vi "UDSSetGenealogy.vi"(8 "Error In":errorcluster, 9 "DataToSet":string[](array[string]), 10 "GenealogyItemsToSet":T1[](array[typedef]), 11 "SessionID":string) -> (0 "Error Out":errorcluster, 2 "Success?":bool)   [LabVIEW 2021, in "Lunar UDS CAN.lvlib"]
uses:
  Lunar UDS CAN.lvlib
  Controls/UDSGenealogyItems.ctl
  Controls/UDSActions.ctl
  abd07550-7e02-4878-985a-2b81226fabe2.vi
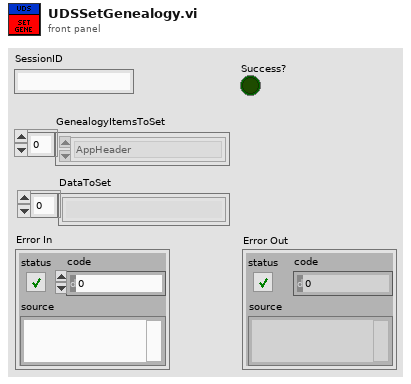
[diagram p1: front panel]
types:
  T1 = typedef "Lunar UDS CAN.lvlib/UDSGenealogyItems.ctl" = enum16{"AppHeader", "Genealogy Block Init", "Genealogy Block", "Board Part Number", "Board Serial Number", "Aux1 Part Number", "Aux1 Serial Number", "Aux2 Part Number", "Aux2 Serial Number", "Config Block Init", "Config Block", "Calibration Block Init", "Calibration Block", "Node Data Block Init", "Node Data Block", "Can Bus Instance"}
  T2 = typedef "Lunar UDS CAN.lvlib/UDSActions.ctl" = enum16{"Open Session", "Connect To Diagnostic Session", "Send Tester Present", "ECU Reset", "Write String Data", "Write Byte Data", "Read Data", "Close Session", "Close All Sessions"}
  T3 = typedef "Lunar UDS CAN.lvlib/UDSGenealoogyItemData.ctl" = cluster{"ID":i32, "ReadOnly":bool, "WriteOnly":bool, "Register Size":i32}
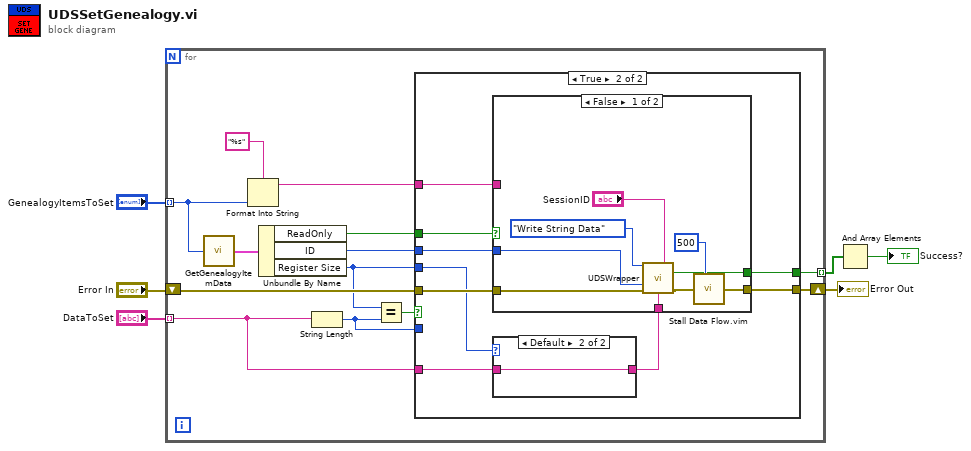
[diagram p0: block diagram]
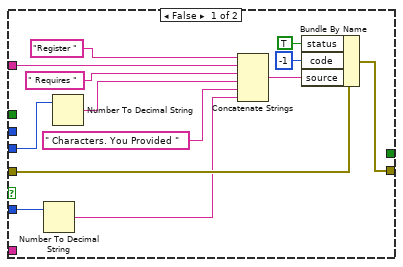
[diagram p2: hidden frame]
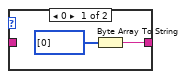
[diagram p3: hidden frame]
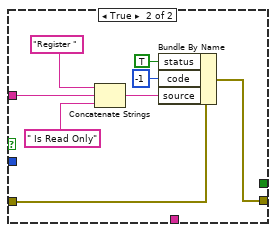
[diagram p4: hidden frame]
diagram:
  n1 = for {
    tunnel: "GenealogyItemsToSet" -> [w12] mode=indexing
    tunnel: "DataToSet" -> [w14] mode=indexing
    shift-right: [w13] -> w3
    shift-left: "Error In" -> [w16]
    tunnel: [w7] -> w2 mode=indexing
    n2 = call "GetGenealogyItemData.vi"("Genealogy Item"=w12) -> ("GenealogyItemData"=w19:T3)
    n3 = Format Into String(format string="%s" ("string (\"\")"), w12) -> (resulting string=w10:string)  [unwired: 2 in, 1 out]
    n4 = Unbundle By Name(w19) -> ("ReadOnly"=w18:bool, "ID"=w17:i32, "Register Size"=w9:i32)
    n5 = String Length(string=w14) -> (length=w8:i32)
    n6 = Equal?(x=w9, y=w8) -> (x = y?=w15:bool)
    n7 = case shown="True" w15 {
      tunnel: w18 -> [_ w41]
      tunnel: w17 -> [_ w40]
      tunnel: w16 -> [w26 w39]
      tunnel: w14 -> [_ w35]
      tunnel: [w27 w38] -> w13
      tunnel: w10 -> [w25 w37]
      tunnel: w9 -> [w24 w36]
      tunnel: w8 -> [w21 _]
      tunnel: [_ w33] -> w7
      frame False {
        n8 = Number To Decimal String(number=w21) -> (decimal integer string=w20:string)  [unwired: 1 in]
        n9 = Number To Decimal String(number=w24) -> (decimal integer string=w23:string)  [unwired: 1 in]
        n10 = Concatenate Strings("Register " ("string"), w25, " Requires " ("string"), w23, " Characters. You Provided " ("string"), w20) -> (w32:string)
        n11 = Bundle By Name(cluster=w26, "status"=TRUE, "code"=-1, "source"=w32) -> (w27:errorcluster)
      }
      frame True {
        n12 = case shown="Default" w36 {
          tunnel: w35 -> [_ w44]
          tunnel: [w42 w44] -> w34
          frame 0 {
            n13 = Byte Array To String(unsigned byte array=u8[] [0]) -> (string=w42:string)
          }
          frame Default {
          }
        }
        n14 = case shown="False" w41 {
          tunnel: w40 -> [w51 _]
          tunnel: w39 -> [w52 w60]
          tunnel: w34 -> [w50 _]
          tunnel: [w48 w61] -> w38
          tunnel: w37 -> [_ w55]
          tunnel: [w46 _] -> w33
          frame False {
            n15 = call "UDSWrapper.vi"("UDS Action"=UDSActions."Write String Data", "SessionID"="SessionID", "ID"=w51, "error in (no error)"=w52, "String Data To Write"=w50) -> ("Success ?"=w46:bool, "error out"=w49:errorcluster)  [unwired: 8 in, 1 out]
            n16 = call "Stall Data Flow.vim"("value in"=w49, "milliseconds to wait"=u32 500) -> ("value out"=w48:errorcluster)  [unwired: 1 out]
          }
          frame True {
            n17 = Concatenate Strings("Register " ("string"), w55, " Is Read Only" ("string")) -> (w57:string)
            n18 = Bundle By Name(cluster=w60, "status"=TRUE, "code"=-1, "source"=w57) -> (w61:errorcluster)
          }
        }
      }
    }
  }
  "Error Out" <- w3
  n19 = And Array Elements(Boolean array=w2) -> (logical AND=→"Success?":bool)
